vi "string to key-value pairs.vi"(4 "separator between key-value pairs":string[](array[string])=[";"], 5 "separator between key and value":string[](array[string])=[":"], 6 "known key list":string[](array[string])=["SET_PID", "SET_OUTPUT"], 7 "input string":string) -> (1 "key index list":i32[](array[numeric]), 2 "value list":string[](array[string]), 3 "key list":string[](array[string]))   [LabVIEW 2016]
uses:
  <vilib>/Utility/error.llb/whitespace.ctl
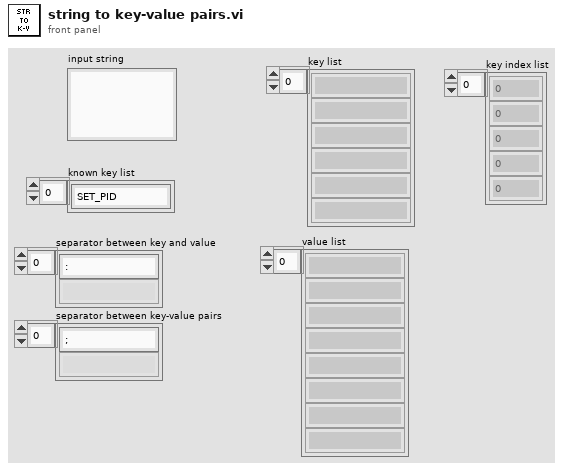
[diagram p1: front panel]
types:
  T1 = typedef "whitespace.ctl" = u16
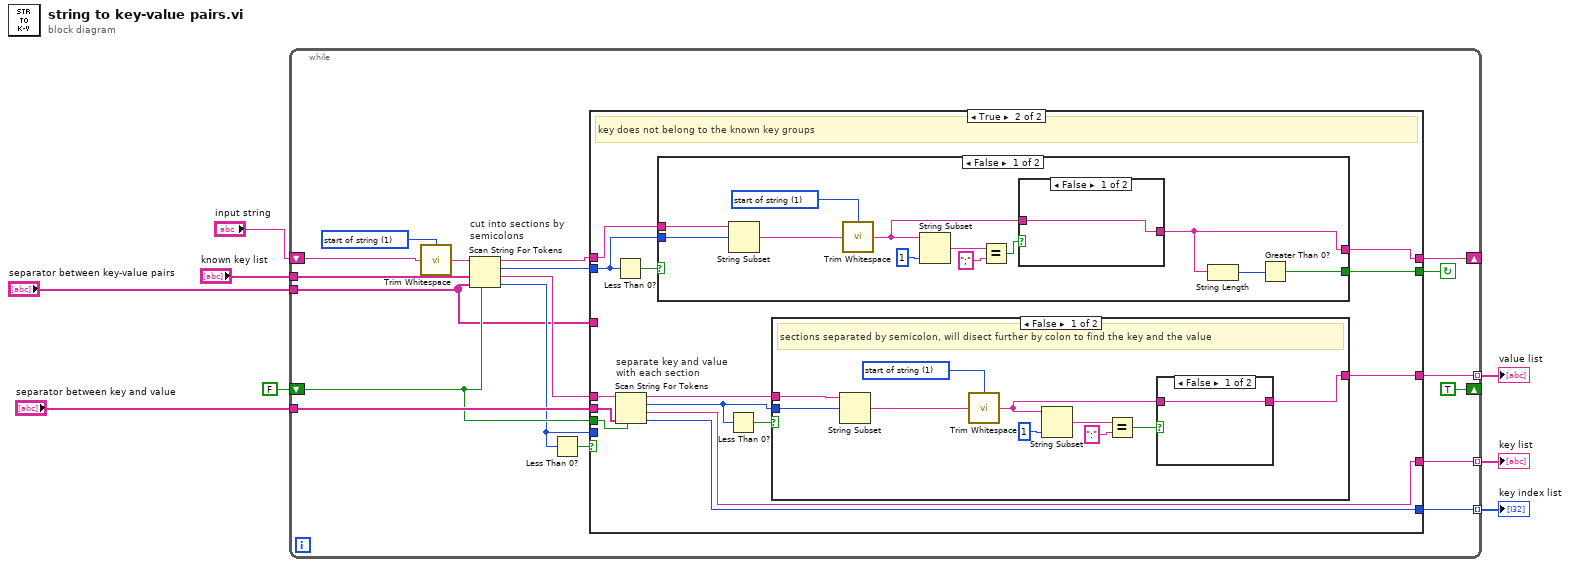
[diagram p0: block diagram]
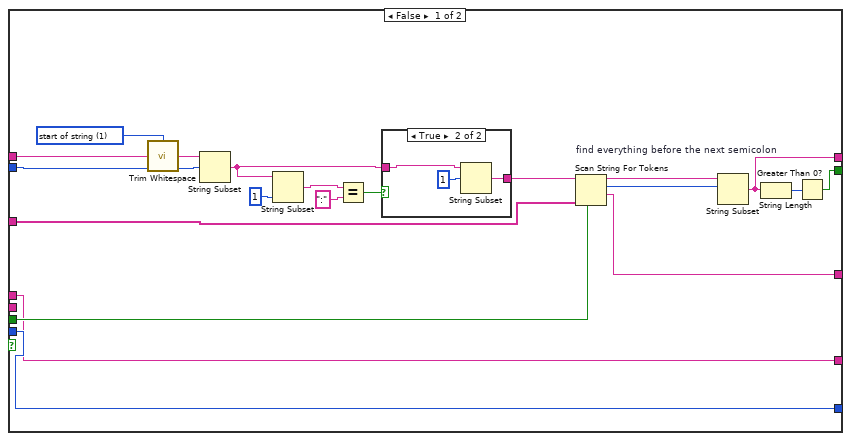
[diagram p2: hidden frame]
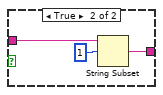
[diagram p4: hidden frame]
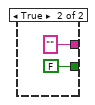
[diagram p5: hidden frame]
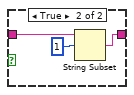
[diagram p6: hidden frame]
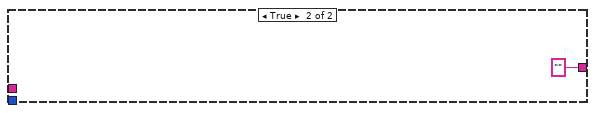
[diagram p7: hidden frame]
diagram:
  n1 = while {
    tunnel: "separator between key-value pairs" -> [w9]
    tunnel: [w22] -> w8 mode=indexing
    tunnel: [w21] -> w7 mode=indexing
    shift-right: [w20] -> _
    shift-left: "input string" -> [w17]
    tunnel: "known key list" -> [w26]
    tunnel: "separator between key and value" -> [w24]
    tunnel: [w19] -> w5 mode=indexing
    shift-right: [TRUE ("use cached delim/oper data? (F)")] -> _
    shift-left: FALSE ("use cached delim/oper data? (F)") -> [w14]
    stop <- w18 continue-if-true
    w15 = T1 1 items=["both", "start of string", "end of string"] ("location (both)")
    n2 = call <vilib>:"Trim Whitespace.vi"("string"=w17, "location (both)"=w15) -> ("trimmed string"=w16:string)
    n3 = Scan String For Tokens "cut into sections by semicolons"(4:w14, 6:w9, 7:w26, 9:w16) -> (0:w10:i32, 1:w23:string, 2:w13:i32, 3:w25:string)  [unwired: 2 in]
    n4 = Less Than 0?(x=w10) -> (x < 0?=w11:bool)
    n5 = case shown="True" w11 {
      tunnel: w25 -> [w45 w64]
      tunnel: w24 -> [_ w63]
      tunnel: w23 -> [w28 w62]
      tunnel: [w28 w61] -> w22
      tunnel: [w46 w60] -> w21
      tunnel: [w31 w58] -> w20
      tunnel: [w34 w57] -> w19
      tunnel: [w29 w56] -> w18
      tunnel: w14 -> [w35 w53]
      tunnel: w13 -> [w27 w51]
      tunnel: w10 -> [w46 _]
      tunnel: w9 -> [w36 _]
      frame False {
        w40 = T1 1 items=["both", "start of string", "end of string"] ("location (both)")
        n6 = call <vilib>:"Trim Whitespace.vi"("string"=w45, "location (both)"=w40) -> ("trimmed string"=w41:string)
        n7 = String Subset(string=w41, offset (0)=w27) -> (substring=w38:string)  [unwired: 1 in]
        n8 = String Subset(string=w38, length (rest)=1 ("length (rest)")) -> (substring=w43:string)  [unwired: 1 in]
        n9 = Equal?(x=w43, y=":") -> (x = y?=w39:bool)
        n10 = case shown="True" w39 {
          tunnel: w38 -> [w47 w50]
          tunnel: [w47 w48] -> w37
          frame False {
          }
          frame True {
            n11 = String Subset(string=w50, offset (0)=1) -> (substring=w48:string)  [unwired: 1 in]
          }
        }
        n12 = Scan String For Tokens "find everything before the next semicolon"(4:w35, 6:w36, 9:w37) -> (1:w34:string, 2:w32:i32, 3:w33:string)  [unwired: 3 in, 1 out]
        n13 = String Subset(string=w33, offset (0)=w32) -> (substring=w31:string)  [unwired: 1 in]
        n14 = String Length(string=w31) -> (length=w30:i32)
        n15 = Greater Than 0?(x=w30) -> (x > 0?=w29:bool)
      }
      frame True {
        # "key does not belong to the known key groups"
        n16 = Less Than 0?(x=w51) -> (x < 0?=w54:bool)
        n17 = Scan String For Tokens "separate key and value with each section"(4:w53, 6:w63, 9:w62) -> (0:w60:i32, 1:w61:string, 2:w52:i32, 3:w59:string)  [unwired: 3 in]
        n18 = case shown="False" w54 {
          tunnel: w64 -> [w76 _]
          tunnel: [w69 "" ("trimmed string")] -> w58
          tunnel: [w67 FALSE] -> w56
          tunnel: w51 -> [w65 _]
          frame False {
            w66 = T1 1 items=["both", "start of string", "end of string"] ("location (both)")
            n19 = String Subset(string=w76, offset (0)=w65) -> (substring=w75:string)  [unwired: 1 in]
            n20 = call <vilib>:"Trim Whitespace.vi"("string"=w75, "location (both)"=w66) -> ("trimmed string"=w70:string)
            n21 = String Subset(string=w70, length (rest)=1 ("length (rest)")) -> (substring=w73:string)  [unwired: 1 in]
            n22 = Equal?(x=w73, y=";") -> (x = y?=w71:bool)
            n23 = case shown="False" w71 {
              tunnel: w70 -> [w77 w80]
              tunnel: [w77 w78] -> w69
              frame False {
              }
              frame True {
                n24 = String Subset(string=w80, offset (0)=1) -> (substring=w78:string)  [unwired: 1 in]
              }
            }
            n25 = String Length(string=w69) -> (length=w68:i32)
            n26 = Greater Than 0?(x=w68) -> (x > 0?=w67:bool)
          }
          frame True {
          }
        }
        n27 = Less Than 0?(x=w52) -> (x < 0?=w55:bool)
        n28 = case shown="False" w55 {
          tunnel: w59 -> [w92 _]
          tunnel: w52 -> [w91 _]
          tunnel: [w84 "" ("trimmed string")] -> w57
          frame False {
            w83 = T1 1 items=["both", "start of string", "end of string"] ("location (both)")
            # "sections separated by semicolon, will disect further by colon to find the key and the value"
            n29 = String Subset(string=w92, offset (0)=w91) -> (substring=w90:string)  [unwired: 1 in]
            n30 = call <vilib>:"Trim Whitespace.vi"("string"=w90, "location (both)"=w83) -> ("trimmed string"=w85:string)
            n31 = String Subset(string=w85, length (rest)=1 ("length (rest)")) -> (substring=w88:string)  [unwired: 1 in]
            n32 = Equal?(x=w88, y=":") -> (x = y?=w86:bool)
            n33 = case shown="False" w86 {
              tunnel: [w93 w95] -> w84
              tunnel: w85 -> [w93 w94]
              frame False {
              }
              frame True {
                n34 = String Subset(string=w94, offset (0)=1) -> (substring=w95:string)  [unwired: 1 in]
              }
            }
          }
          frame True {
          }
        }
      }
    }
  }
  "value list" <- w5
  "key list" <- w8
  "key index list" <- w7
